vi "FTW-Consumer-Worker.vi"(1 "Endpoint":refnum<class "FTW-Endpoint.lvclass">, 2 "Message Handler":refnum<user-event>) -> ()   [LabVIEW 2013, in "FTW-Consumer.lvclass"]
uses:
  FTW-Consumer.lvclass
  Message/Base/FTW-Message.lvclass
  Endpoint/FTW-Endpoint.lvclass
panel:
  out "Messages Handled":u32
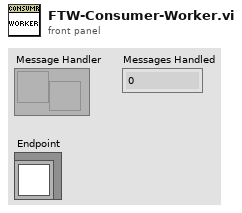
[diagram p1: front panel]
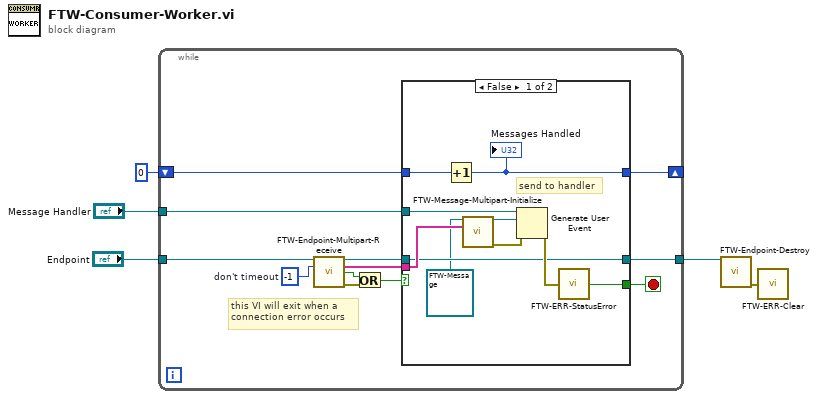
[diagram p0: block diagram]
diagram:
  n1 = while {
    tunnel: "Message Handler" -> [w17]
    shift-right: [w10] -> _
    shift-left: u32 0 -> [w11]
    tunnel: "Endpoint" -> [w16]
    tunnel: [w6] -> w3
    stop <- w12 stop-if-true
    w15 = -1  # don't timeout
    # "this VI will exit when a\nconnection error occurs"
    n2 = call-dynamic "FTW-Endpoint-Multipart-Receive.vi"("FTW Endpoint"=w16, "Timeout"=w15) -> ("FTW Endpoint out"=w9:refnum<class "FTW-Endpoint.lvclass">, "Message Received"=w13:string[], "Timed out?"=w7:bool, "error out"=w14:errorcluster)  [unwired: 10 in]
    n3 = Or(x=w7, y=w14) -> (x .or. y?=w8:bool)
    n4 = case shown="False" w8 {
      tunnel: w17 -> [w27 _]
      tunnel: w13 -> [w24 _]
      tunnel: [w23 TRUE] -> w12
      tunnel: w9 -> [w22 w28]
      tunnel: w11 -> [w26 w30]
      tunnel: [w21 w30] -> w10
      tunnel: [w22 w28] -> w6
      frame False {
        # "send to handler"
        n5 = Increment(x=w26) -> (x+1=w21:u32)
        "Messages Handled" <- w21
        n6 = call-dynamic "FTW-Message-Multipart-Initialize.vi"("FTW Message"=refnum<class "FTW-Message.lvclass"> refnum, "Message Parts"=w24) -> ("FTW Message out"=w19:refnum<class "FTW-Message.lvclass">, "error out"=w20:errorcluster)  [unwired: 12 in]
        n7 = Generate User Event(user event=w27, event data cluster=w19, error in=w20) -> (error out=w25:errorcluster)  [unwired: 1 in, 1 out]
        n8 = call "FTW-ERR-StatusError.vi"("error to check"=w25) -> ("Error?"=w23:bool)
      }
      frame True {
        # "did not get a message in time\nor receive errored"
      }
    }
  }
  n9 = call-dynamic "FTW-Endpoint-Destroy.vi"("FTW Endpoint"=w3) -> ("error out"=w1:errorcluster)  [unwired: 14 in]
  n10 = call "FTW-ERR-Clear.vi"("error to snuff"=w1) -> ()  [unwired: 1 out]
